vi "Merge_row_values.vi"(2 "Present Row values":string[](array[string]), 3 "Present Channels":string[](array[string]), 4 "Desired Channels":string[](array[string])) -> (1 "Desired Row values":string[](array[string]))   [LabVIEW 2010]
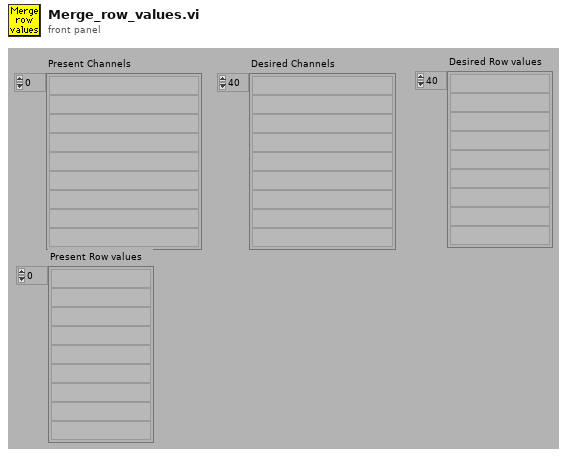
[diagram p1: front panel]
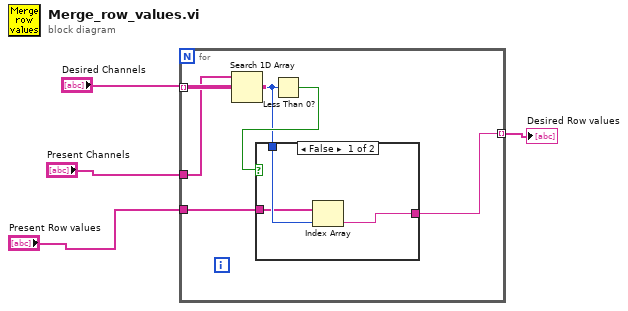
[diagram p0: block diagram]
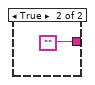
[diagram p2: hidden frame]
diagram:
  n1 = for {
    tunnel: "Present Channels" -> [w10]
    tunnel: "Desired Channels" -> [w9] mode=indexing
    tunnel: "Present Row values" -> [w7]
    tunnel: [w6] -> w4 mode=indexing
    n2 = Search 1D Array(1D array=w10, element=w9) -> (index of element=w5:i32)  [unwired: 1 out]
    n3 = Less Than 0?(x=w5) -> (x < 0?=w8:bool)
    n4 = case shown="False" w8 {
      tunnel: w5 -> [w13 _]
      tunnel: w7 -> [w12 _]
      tunnel: [w11 ""] -> w6
      frame False {
        n5 = Index Array(array=w12, index=w13) -> (element=w11:string)
      }
      frame True {
      }
    }
  }
  "Desired Row values" <- w4
